vi "Clear.vi"(8 "error in (no error)":errorcluster, 11 "TestView_Tree in":refnum<class "TestView_Tree_Single.lvclass">) -> (0 "error out":errorcluster, 3 "TestView_Tree out":refnum<class "TestView_Tree_Single.lvclass">)   [LabVIEW 2022 SP3, in "TestView_Tree_Single.lvlib" / "TestView_Tree_Single.lvclass"]
uses:
  TestView_Tree_Single.lvclass
  Components/TestView_Base.lvlibp/ViewStatus.ctl
  Components/TestView_Base.lvlibp/TestView_Base.lvclass
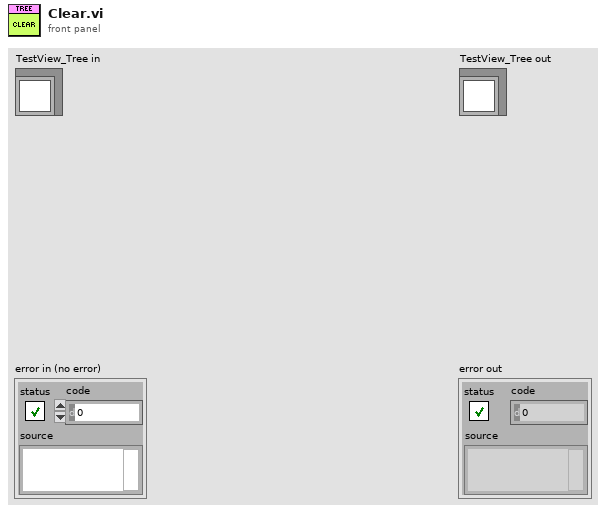
[diagram p1: front panel]
types:
  T1 = typedef "TestView_Base.lvlibp/TestView_Base.lvclass/ViewStatus.ctl" = enum16{"Testing", "Ready", "Logout", "Login", "PASS", "FAIL", "FAULT", "ABORTED"}
  T2 = typedef "TestView_Tree_Single.lvlib/TestView_Tree_Single.lvclass/ObjectAttributes.ctl" = cluster{"Front Panel":refnum<vi>, "Last_Item":string, "Config":T3, "Title":string, "User":string, "TreeRef":refnum<vi>, "Active DUT":i32, "Status":T1, "SN":string, "Spec":string}
  T3 = typedef "TestView_Tree_Single.lvlib/TestView_Tree_Single.lvclass/Config.ctl" = cluster{"default":string}
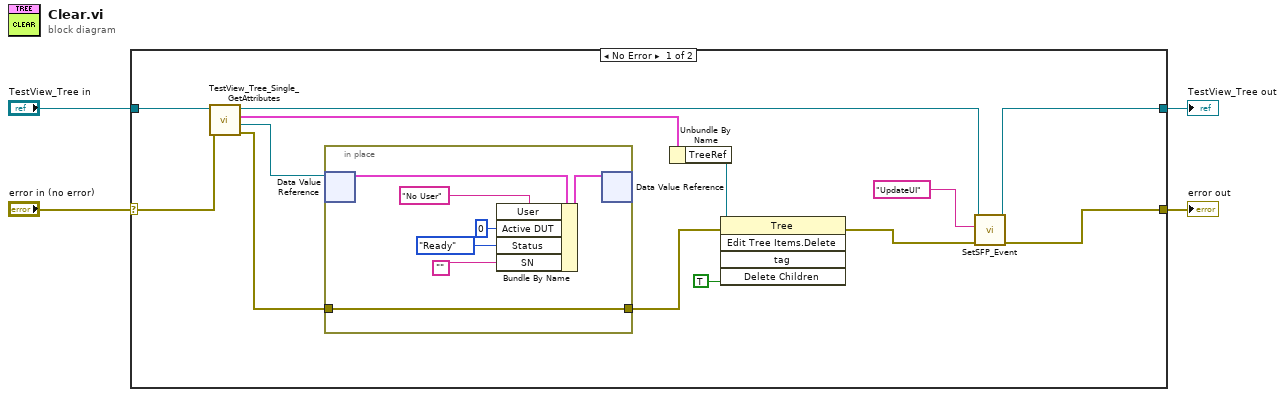
[diagram p0: block diagram]
diagram:
  n1 = case shown="No Error" "error in (no error)" {
    selector: "error in (no error)" -> [w15 w26]
    tunnel: [w7 w26] -> w3
    tunnel: [w5 w25] -> w1
    tunnel: "TestView_Tree in" -> [w16 w25]
    frame No Error {
      n2 = call "TestView_Tree_Single_GetAttributes.vi"("error in (no error)"=w15, "reference in"=w16) -> ("error out"=w11:errorcluster, "DataRef"=w12:refnum<data-value>, "Data"=w14:T2, "reference out"=w6:refnum<class "TestView_Tree_Single.lvclass">)  [unwired: 6 in]
      n3 = in-place {
        in-place-border: w11 -> [w21]
        in-place-border: [w21] -> w10
        n4 = in-place-dvr #1(w12) -> (w23:T2)  [unwired: 1 out]
        n5 = Bundle By Name(cluster=w23, "User"="No User", "Active DUT"=0, "Status"=ViewStatus."Ready", "SN"="") -> (w22:T2)
        n6 = in-place-dvr #1(w22) -> ()  [unwired: 2 out]
      }
      n7 = Unbundle By Name(w14) -> ("TreeRef"=w13:refnum<vi>)
      n8 = invoke class="Tree" method="Edit Tree Items.Delete"(reference=w13, error in=w10, "Delete Children"=TRUE ("Delete Children?")) -> (error out=w8:errorcluster)  [unwired: 2 in, 4 out]
      n9 = call-dynamic "SetSFP_Event.vi"("error in (no error)"=w8, "msg"="UpdateUI", "reference in"=w6) -> ("error out"=w7:errorcluster, "reference out"=w5:refnum<class "TestView_Tree_Single.lvclass">)  [unwired: 7 in]
    }
    frame Error {
    }
  }
  "error out" <- w3
  "TestView_Tree out" <- w1
